vi "BRig_dataExp_FreeReward_Switch.vi"() -> (2 "output_FreeReward_Switch":i32)   [LabVIEW 2014]
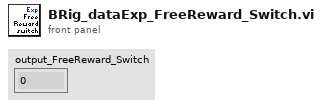
[diagram p1: front panel]
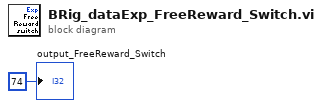
[diagram p0: block diagram]
diagram:
  "output_FreeReward_Switch" <- 74 ("output_iBlock")
